vi "AlliGator Image Contrast Status.vi"(2 "Flag (in)":bool, 4 "Read/Write":T1) -> (7 "Flag (out)":bool)   [LabVIEW 2021, in "AlliGator Source Image.lvlib"]
doc: "Raises the flag when calling the action.\nLowers it when done."
uses:
  AlliGator Source Image.lvlib
  Utilities/Read-Write.ctl
  Utilities/Utilities.lvlib
panel:
  # "see the AlliGator License on the block diagram (Ctrl+E or Window:Show Block Diagram)"
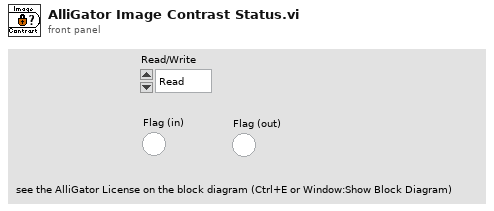
[diagram p1: front panel]
types:
  T1 = typedef "Utilities.lvlib/Read-Write.ctl" = enum16{"Read", "Write"}
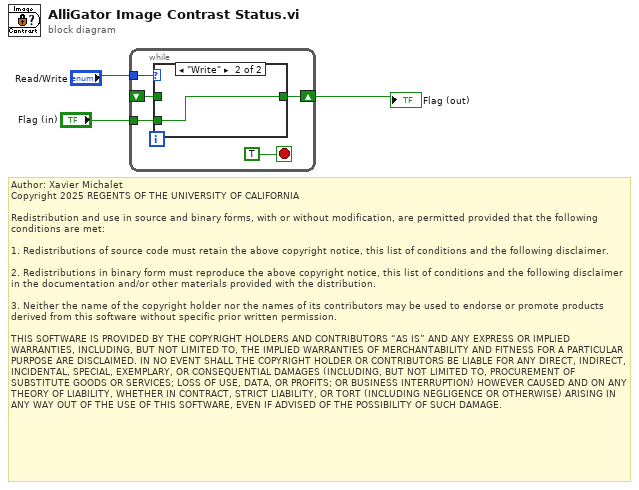
[diagram p0: block diagram]
diagram:
  # "Author: Xavier Michalet\nCopyright 2025 REGENTS OF THE UNIVERSITY OF CALIFORNIA\n\nRedistribution and use in source and binary forms, with or without modification, are permitted provided that the following conditions are met:\n\n1. Redistributions of source code must retain the above copyright notice, this list of conditions and the following disclaimer.\n\n2. Redistributions in binary form must reproduce the above copyright notice, this list of conditions and the following disclaimer in the documentation and/or other materials provided with the distribution.\n\n3. Neither the name of the copyright holder nor the names of its contributors may be used to endorse or promote products derived from this software without specific prior written permission.\n\nTHIS SOFTWARE IS PROVIDED BY THE COPYRIGHT HOLDERS AND CONTRIBUTORS “AS IS” AND ANY EXPRESS OR IMPLIED WARRANTIES, INCLUDING, BUT NOT LIMITED TO, THE IMPLIED WARRANTIES OF MERCHANTABILITY AND FITNESS FOR A PARTICULAR PURPOSE ARE DISCLAIMED. IN NO EVENT SHALL THE COPYRIGHT HOLDER OR CONTRIBUTORS BE LIABLE FOR ANY DIRECT, INDIRECT, INCIDENTAL, SPECIAL, EXEMPLARY, OR CONSEQUENTIAL DAMAGES (INCLUDING, BUT NOT LIMITED TO, PROCUREMENT OF SUBSTITUTE GOODS OR SERVICES; LOSS OF USE, DATA, OR PROFITS; OR BUSINESS INTERRUPTION) HOWEVER CAUSED AND ON ANY THEORY OF LIABILITY, WHETHER IN CONTRACT, STRICT LIABILITY, OR TORT (INCLUDING NEGLIGENCE OR OTHERWISE) ARISING IN ANY WAY OUT OF THE USE OF THIS SOFTWARE, EVEN IF ADVISED OF THE POSSIBILITY OF SUCH DAMAGE."
  n1 = while {
    tunnel: "Read/Write" -> [w7]
    shift-right: [w5] -> w1
    shift-left: _ -> [w6]
    tunnel: "Flag (in)" -> [w4]
    stop <- TRUE stop-if-true
    n2 = case shown="\"Write\"" w7 {
      tunnel: w6 -> [w9 _]
      tunnel: [w9 w10] -> w5
      tunnel: w4 -> [_ w10]
      frame "Read", Default {
      }
      frame "Write" {
      }
    }
  }
  "Flag (out)" <- w1
